vi "iRobot Demo.vi"(8 "error in":errorcluster, 9 "Demo":T2=enum."Banjo", 11 "UART port in":T1) -> (0 "error out":errorcluster, 3 "UART port out":T1)   [LabVIEW 2010]
doc: "Instruct the robot to execute a pre-configured demo.\n\nThis VI writes to, but does not read from, the serial port."
uses:
  Command Controls/iRobot Demo Numbers.ctl
  UART/UART Port Type.ctl
  Open Interface Controls/iRobot OpCode.ctl
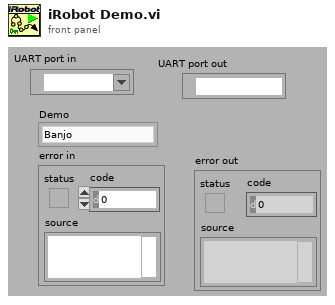
[diagram p1: front panel]
types:
  T1 = typedef "UART Port Type.ctl" = refnum<visa-resource-name>
  T2 = typedef "iRobot Demo Numbers.ctl" = enum8{"Cover", "Cover and Duck", "Spot Cover", "Mouse", "Drive Figure Eight", "Wimp", "Home", "Tag", "Pachelbel", "Banjo"}
  T3 = typedef "iRobot OpCode.ctl" = u8
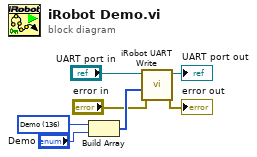
[diagram p0: block diagram]
diagram:
  w7 = T3 136 items=["Start"=128, "Baud"=129, "Control"=130, "Safe"=131, "Full"=132, "Demo"=136, "Demo - Cover"=135, "Demo - Cover and Dock"=143, "Demo - Spot"=134, "Drive"=137, "Drive Direct"=145, "LEDs"=139, "Digital Outputs"=147, "PWM Low Side Drivers"=144, "Low Side Drivers"=138, "Send IR"=151, "Song"=140, "Play Song"=141, "Sensors"=142, "Query List"=149, "Stream"=148, "Pause/Resume Stream"=150, "Script"=152, "Play Script"=153, "Show Script"=154, "Wait Time"=155, "Wait Distance"=156, "Wait Angle"=157, "Wait Event"=158] ("OpCode")
  n1 = Build Array(w7, "Demo") -> (w3:T3[])
  n2 = call "iRobot UART Write.vi"("error in"="error in", "data"=w3, "UART port in"="UART port in") -> ("error out"=→"error out":errorcluster, "UART port out"=→"UART port out":T1)  [unwired: 7 in]
